vi "Parse VI XML - Splitter Style.vi"(5 "Action":T1(ring), 7 "UID":i32=83, 8 "New Style":T2 items=["Modern", "Classic", "System", "NXG"], 9 "VI XML in":string="<SL__rootObject class=\"oHExt\" uid=\"1\">\n  <root class=\"supC\" uid=\"10\">\n    <objFlags>65536</objFlags>\n    <bounds>(0, 0, 0, 0)</bounds>\n    <MouseWheelSupport>0</MouseWheelSupport>\n    <ddoList elements=\"1\">\n      <SL__arrayElement uid=\"206\"/>\n      </ddoList>\n    <paneHierarchy class=\"splitter\" uid=\"83\">\n      <objFlags>393232</objFlags>\n      <bounds>(46, 0, 434, 621)</bounds>\n      <partsList elements=\"3\">\n        <SL__arrayElement class=\"label\" uid=\"90\">\n          <objFlags>1511754</objFlags>\n          <partID>16</partID>\n          <masterPart>102</masterPart>\n          <howGrow>4108</howGrow>\n          <bounds>(133, 231, 255, 241)</bounds>\n          <image class=\"Image\">\n            <ImageResID>-9</ImageResID>\n            </image>\n          <fgColor>01000000</fgColor>\n          <bgColor>01000000</bgColor>\n          <textRec class=\"textHair\">\n            <mode>1029</mode>\n            <text>\"Splitter\"</text>\n            <bgColor>01000000</bgColor>\n            </textRec>\n          </SL__arrayElement>\n        <SL__arrayElement class=\"bigMultiCosm\" uid=\"91\">\n          <objFlags>2320</objFlags>\n          <partID>102</partID>\n          <bounds>(0, 228, 388, 234)</bounds>\n          <fgColor>00BCBCBC</fgColor>\n          <bgColor>00BCBCBC</bgColor>\n          <index>1</index>\n          <table elements=\"3\">\n            <SL__arrayElement class=\"SubCosm\">\n              <Bounds>(0, 0, 388, 6)</Bounds>\n              <FGColor>00BCBCBC</FGColor>\n              <BGColor>00BCBCBC</BGColor>\n              <Image class=\"Image\">\n                <ImageResID>-428</ImageResID>\n                </Image>\n              </SL__arrayElement>\n            <SL__arrayElement class=\"SubCosm\">\n              <Bounds>(0, 0, 388, 6)</Bounds>\n              <FGColor>00BCBCBC</FGColor>\n              <BGColor>00BCBCBC</BGColor>\n              <Image class=\"Image\">\n                <ImageResID>-11</ImageResID>\n                </Image>\n              </SL__arrayElement>\n            <SL__arrayElement class=\"SubCosm\">\n              <Bounds>(0, 0, 388, 6)</Bounds>\n              <FGColor>01000016</FGColor>\n              <BGColor>01000016</BGColor>\n              <Image class=\"Image\">\n                <ImageResID>-9</ImageResID>\n                </Image>\n              </SL__arrayElement>\n            </table>\n          </SL__arrayElement>\n        <SL__arrayElement class=\"annex\" uid=\"92\">\n          <partID>66</partID>\n          <refListLength>0</refListLength>\n          <hGrowNodeListLength>1</hGrowNodeListLength>\n          </SL__arrayElement>\n        </partsList>\n      <topOrLeft class=\"pane\" uid=\"104\">\n        <objFlags>2492464</objFlags>\n        <bounds>(0, 0, 388, 228)</bounds>\n        <partsList elements=\"6\">\n          <SL__arrayElement class=\"label\" uid=\"107\">\n            <objFlags>1511754</objFlags>\n            <partID>16</partID>\n            <masterPart>28</masterPart>\n            <howGrow>5</howGrow>\n            <bounds>(0, 0, 17, 29)</bounds>\n            <image class=\"Image\">\n              <ImageResID>-9</ImageResID>\n              </image>\n            <fgColor>01000000</fgColor>\n            <bgColor>01000000</bgColor>\n            <textRec class=\"textHair\">\n              <mode>1028</mode>\n              <text>\"Pane\"</text>\n              <bgColor>01000000</bgColor>\n              </textRec>\n            </SL__arrayElement>\n          <SL__arrayElement class=\"cosm\" uid=\"108\">\n            <objFlags>3442</objFlags>\n            <partID>39</partID>\n            <masterPart>28</masterPart>\n            <howGrow>194</howGrow>\n            <bounds>(0, 211, 371, 228)</bounds>\n            <image class=\"Image\">\n              <ImageResID>0</ImageResID>\n              </image>\n            <bgColor>00B3B3B3</bgColor>\n            </SL__arrayElement>\n          <SL__arrayElement class=\"cosm\" uid=\"109\">\n            <objFlags>3442</objFlags>\n            <partID>38</partID>\n            <masterPart>28</masterPart>\n            <howGrow>56</howGrow>\n            <bounds>(371, 0, 388, 211)</bounds>\n            <image class=\"Image\">\n              <ImageResID>0</ImageResID>\n              </image>\n            <bgColor>00B3B3B3</bgColor>\n            </SL__arrayElement>\n          <SL__arrayElement class=\"cosm\" uid=\"110\">\n            <objFlags>3443</objFlags>\n            <partID>44</partID>\n            <masterPart>28</masterPart>\n            <howGrow>10</howGrow>\n            <bounds>(371, 211, 388, 228)</bounds>\n            <image class=\"Image\">\n              <ImageResID>-365</ImageResID>\n              </image>\n            <fgColor>00B3B3B3</fgColor>\n            <bgColor>00B3B3B3</bgColor>\n            </SL__arrayElement>\n          <SL__arrayElement class=\"cosm\" uid=\"111\">\n            <objFlags>115</objFlags>\n            <partID>28</partID>\n            <howGrow>120</howGrow>\n            <bounds>(0, 0, 371, 211)</bounds>\n            <image class=\"Image\">\n              <ImageResID>-704</ImageResID>\n              </image>\n            <fgColor>00E2E2E2</fgColor>\n            <bgColor>00E2E2E2</bgColor>\n            </SL__arrayElement>\n          <SL__arrayElement class=\"annex\" uid=\"112\">\n            <partID>66</partID>\n            </SL__arrayElement>\n          </partsList>\n        <paneFlags>331089</paneFlags>\n        <minPaneSize>(1,1)</minPaneSize>\n        <docBounds>(-138, 0, 325, 232)</docBounds>\n        <zPlaneList elements=\"1\">\n          <SL__arrayElement class=\"fPDCO\" uid=\"206\">\n            <objFlags>1</objFlags>\n            <typeDesc>TypeID(1)</typeDesc>\n            <ddo class=\"stdNum\" uid=\"190\">\n              <objFlags>393217</objFlags>\n              <bounds>(0, 105, 41, 180)</bounds>\n              <partsList elements=\"8\">\n                <SL__arrayElement class=\"label\" uid=\"196\">\n                  <objFlags>1507654</objFlags>\n                  <partID>16</partID>\n                  <masterPart>9</masterPart>\n                  <howGrow>4096</howGrow>\n                  <bounds>(0, 0, 17, 22)</bounds>\n                  <image class=\"Image\">\n                    <ImageResID>-9</ImageResID>\n                    </image>\n                  <fgColor>01000000</fgColor>\n                  <bgColor>01000000</bgColor>\n                  <textRec class=\"textHair\">\n                    <flags>512</flags>\n                    <mode>17412</mode>\n                    <text>\"UID\"</text>\n                    <bgColor>01000000</bgColor>\n                    </textRec>\n                  </SL__arrayElement>\n                <SL__arrayElement class=\"numLabel\" uid=\"197\">\n                  <objFlags>264498</objFlags>\n                  <partID>10</partID>\n                  <masterPart>9</masterPart>\n                  <howGrow>240</howGrow>\n                  <bounds>(19, 2, 39, 74)</bounds>\n                  <image class=\"Image\">\n                    <ImageResID>-2002</ImageResID>\n                    </image>\n                  <fgColor>00FFFFFF</fgColor>\n                  <bgColor>00E8EBED</bgColor>\n                  <textRec class=\"textHair\">\n                    <flags>1536</flags>\n                    <mode>8389650</mode>\n                    <view>(1, 0, -2, 0)</view>\n                    <bgColor>00E8EBED</bgColor>\n                    </textRec>\n                  <format>\"%25.0f\"</format>\n                  </SL__arrayElement>\n                <SL__arrayElement class=\"bigMultiCosm\" uid=\"198\">\n                  <objFlags>6458</objFlags>\n                  <partID>2</partID>\n                  <masterPart>9</masterPart>\n                  <howGrow>2054</howGrow>\n                  <bounds>(17, 62, 28, 75)</bounds>\n                  <fgColor>002B3033</fgColor>\n                  <bgColor>00A8ABAE</bgColor>\n                  <table elements=\"2\">\n                    <SL__arrayElement class=\"SubCosm\">\n                      <Bounds>(0, 0, 11, 13)</Bounds>\n                      <FGColor>002B3033</FGColor>\n                      <BGColor>00A8ABAE</BGColor>\n                      <Image class=\"Image\">\n                        <ImageResID>-774</ImageResID>\n                        </Image>\n                      </SL__arrayElement>\n                    <SL__arrayElement class=\"SubCosm\">\n                      <Bounds>(0, 0, 11, 13)</Bounds>\n                      <FGColor>002B3033</FGColor>\n                      <BGColor>004384B7</BGColor>\n                      <Image class=\"Image\">\n                        <ImageResID>-774</ImageResID>\n                        </Image>\n                      </SL__arrayElement>\n                    </table>\n                  </SL__arrayElement>\n                <SL__arrayElement class=\"bigMultiCosm\" uid=\"199\">\n                  <objFlags>6458</objFlags>\n                  <partID>3</partID>\n                  <masterPart>9</masterPart>\n                  <howGrow>1034</howGrow>\n                  <bounds>(30, 62, 41, 75)</bounds>\n                  <fgColor>002B3033</fgColor>\n                  <bgColor>00A8ABAE</bgColor>\n                  <table elements=\"2\">\n                    <SL__arrayElement class=\"SubCosm\">\n                      <Bounds>(0, 0, 11, 13)</Bounds>\n                      <FGColor>002B3033</FGColor>\n                      <BGColor>00A8ABAE</BGColor>\n                      <Image class=\"Image\">\n                        <ImageResID>-775</ImageResID>\n                        </Image>\n                      </SL__arrayElement>\n                    <SL__arrayElement class=\"SubCosm\">\n                      <Bounds>(0, 0, 11, 13)</Bounds>\n                      <FGColor>002B3033</FGColor>\n                      <BGColor>004384B7</BGColor>\n                      <Image class=\"Image\">\n                        <ImageResID>-775</ImageResID>\n                        </Image>\n                      </SL__arrayElement>\n                    </table>\n                  </SL__arrayElement>\n                <SL__arrayElement class=\"multiCosm\" uid=\"200\">\n                  <objFlags>6458</objFlags>\n                  <partID>15</partID>\n                  <masterPart>9</masterPart>\n                  <howGrow>13</howGrow>\n                  <bounds>(22, 1, 37, 7)</bounds>\n                  <fgColor>002B3033</fgColor>\n                  <bgColor>00DBDFE2</bgColor>\n                  <table elements=\"5\">\n                    <SL__arrayElement class=\"Image\">\n                      <ImageResID>-2000</ImageResID>\n                      </SL__arrayElement>\n                    <SL__arrayElement class=\"Image\">\n                      <ImageResID>-2001</ImageResID>\n                      </SL__arrayElement>\n                    <SL__arrayElement class=\"Image\">\n                      <ImageResID>-2002</ImageResID>\n                      </SL__arrayElement>\n                    <SL__arrayElement class=\"Image\">\n                      <ImageResID>-2003</ImageResID>\n                      </SL__arrayElement>\n                    <SL__arrayElement class=\"Image\">\n                      <ImageResID>-2095</ImageResID>\n                      </SL__arrayElement>\n                    </table>\n                  </SL__arrayElement>\n                <SL__arrayElement class=\"multiCosm\" uid=\"201\">\n                  <objFlags>6462</objFlags>\n                  <partID>118</partID>\n                  <masterPart>9</masterPart>\n                  <howGrow>193</howGrow>\n                  <bounds>(18, 1, 40, 7)</bounds>\n                  <fgColor>00DBDFE2</fgColor>\n                  <bgColor>00DBDFE2</bgColor>\n                  <table elements=\"5\">\n                    <SL__arrayElement class=\"Image\">\n                      <ImageResID>-11</ImageResID>\n                      </SL__arrayElement>\n                    <SL__arrayElement class=\"Image\">\n                      <ImageResID>-11</ImageResID>\n                      </SL__arrayElement>\n                    <SL__arrayElement class=\"Image\">\n                      <ImageResID>-11</ImageResID>\n                      </SL__arrayElement>\n                    <SL__arrayElement class=\"Image\">\n                      <ImageResID>-11</ImageResID>\n                      </SL__arrayElement>\n                    <SL__arrayElement class=\"Image\">\n                      <ImageResID>-11</ImageResID>\n                      </SL__arrayElement>\n                    </table>\n                  </SL__arrayElement>\n                <SL__arrayElement class=\"cosm\" uid=\"202\">\n                  <objFlags>2327</objFlags>\n                  <partID>9</partID>\n                  <howGrow>240</howGrow>\n                  <bounds>(17, 0, 41, 75)</bounds>\n                  <image class=\"Image\">\n                    <ImageResID>-786</ImageResID>\n                    </image>\n                  <fgColor>00A8ABAE</fgColor>\n                  <bgColor>00E8EBED</bgColor>\n                  </SL__arrayElement>\n                <SL__arrayElement class=\"annex\" uid=\"203\">\n                  <partID>66</partID>\n                  <refListLength>0</refListLength>\n                  <hGrowNodeListLength>0</hGrowNodeListLength>\n                  <rsrcID>32707</rsrcID>\n                  </SL__arrayElement>\n                </partsList>\n              <typeDesc>TypeID(2)</typeDesc>\n              <MouseWheelSupport>2</MouseWheelSupport>\n              <StdNumMin>-2147483648</StdNumMin>\n              <StdNumMax>2147483647</StdNumMax>\n              <StdNumInc>0</StdNumInc>\n              </ddo>\n            <conNum>-1</conNum>\n            <termListLength>1</termListLength>\n            </SL__arrayElement>\n          </zPlaneList>\n        <image class=\"Image\">\n          <ImageResID>0</ImageResID>\n          </image>\n        </topOrLeft>\n      <botOrRight class=\"pane\" uid=\"95\">\n        <objFlags>2492464</objFlags>\n        <bounds>(0, 234, 388, 621)</bounds>\n        <partsList elements=\"6\">\n          <SL__arrayElement class=\"label\" uid=\"98\">\n            <objFlags>1511754</objFlags>\n            <partID>16</partID>\n            <masterPart>28</masterPart>\n            <howGrow>5</howGrow>\n            <bounds>(0, 0, 17, 38)</bounds>\n            <image class=\"Image\">\n              <ImageResID>-9</ImageResID>\n              </image>\n            <fgColor>01000000</fgColor>\n            <bgColor>01000000</bgColor>\n            <textRec class=\"textHair\">\n              <mode>1028</mode>\n              <text>\"Pane 2\"</text>\n              <bgColor>01000000</bgColor>\n              </textRec>\n            </SL__arrayElement>\n          <SL__arrayElement class=\"cosm\" uid=\"99\">\n            <objFlags>3442</objFlags>\n            <partID>39</partID>\n            <masterPart>28</masterPart>\n            <howGrow>194</howGrow>\n            <bounds>(0, 370, 371, 387)</bounds>\n            <image class=\"Image\">\n              <ImageResID>0</ImageResID>\n              </image>\n            <bgColor>00B3B3B3</bgColor>\n            </SL__arrayElement>\n          <SL__arrayElement class=\"cosm\" uid=\"100\">\n            <objFlags>3442</objFlags>\n            <partID>38</partID>\n            <masterPart>28</masterPart>\n            <howGrow>56</howGrow>\n            <bounds>(371, 0, 388, 370)</bounds>\n            <image class=\"Image\">\n              <ImageResID>0</ImageResID>\n              </image>\n            <bgColor>00B3B3B3</bgColor>\n            </SL__arrayElement>\n          <SL__arrayElement class=\"cosm\" uid=\"101\">\n            <objFlags>3443</objFlags>\n            <partID>44</partID>\n            <masterPart>28</masterPart>\n            <howGrow>10</howGrow>\n            <bounds>(371, 370, 388, 387)</bounds>\n            <image class=\"Image\">\n              <ImageResID>-365</ImageResID>\n              </image>\n            <fgColor>00B3B3B3</fgColor>\n            <bgColor>00B3B3B3</bgColor>\n            </SL__arrayElement>\n          <SL__arrayElement class=\"cosm\" uid=\"102\">\n            <objFlags>115</objFlags>\n            <partID>28</partID>\n            <howGrow>120</howGrow>\n            <bounds>(0, 0, 371, 370)</bounds>\n            <image class=\"Image\">\n              <ImageResID>-704</ImageResID>\n              </image>\n            <fgColor>00E2E2E2</fgColor>\n            <bgColor>00E2E2E2</bgColor>\n            </SL__arrayElement>\n          <SL__arrayElement class=\"annex\" uid=\"103\">\n            <partID>66</partID>\n            </SL__arrayElement>\n          </partsList>\n        <paneFlags>331089</paneFlags>\n        <minPaneSize>(1,1)</minPaneSize>\n        <docBounds>(-46, 0, 325, 370)</docBounds>\n        <zPlaneList elements=\"0\">\n          </zPlaneList>\n        <image class=\"Image\">\n          <ImageResID>0</ImageResID>\n          </image>\n        </botOrRight>\n      <splitterFlags>1</splitterFlags>\n      <ratio>3.671498E-1 (%x0EFBBB3E)</ratio>\n      </paneHierarchy>\n    <savedSize>(0, 0, 0, 0)</savedSize>\n    <conPane class=\"conPane\" uid=\"21\">\n      <conId>4815</conId>\n      <cons elements=\"12\">\n        </cons>\n      </conPane>\n    <keyMappingList class=\"keyMapList\" uid=\"22\">\n      </keyMappingList>\n    </root>\n  <pBounds>(46, 0, 434, 621)</pBounds>\n  <dBounds>(0, 0, 0, 0)</dBounds>\n  <origin>(435,189)</origin>\n  <instrStyle>31</instrStyle>\n  <blinkList elements=\"0\">\n    </blinkList>\n  </SL__rootObject>\n") -> (2 "Old Style":T2 items=["Modern", "Classic", "System", "NXG"], 3 "VI XML out":string="<SL__rootObject class=\"oHExt\" uid=\"1\">\n  <root class=\"supC\" uid=\"10\">\n    <objFlags>65536</objFlags>\n    <bounds>(0, 0, 0, 0)</bounds>\n    <MouseWheelSupport>0</MouseWheelSupport>\n    <ddoList elements=\"1\">\n      <SL__arrayElement uid=\"206\"/>\n      </ddoList>\n    <paneHierarchy class=\"splitter\" uid=\"83\">\n      <objFlags>393232</objFlags>\n      <bounds>(46, 0, 434, 621)</bounds>\n      <partsList elements=\"3\">\n        <SL__arrayElement class=\"label\" uid=\"90\">\n          <objFlags>1511754</objFlags>\n          <partID>16</partID>\n          <masterPart>102</masterPart>\n          <howGrow>4108</howGrow>\n          <bounds>(133, 231, 255, 241)</bounds>\n          <image class=\"Image\">\n            <ImageResID>-9</ImageResID>\n            </image>\n          <fgColor>01000000</fgColor>\n          <bgColor>01000000</bgColor>\n          <textRec class=\"textHair\">\n            <mode>1029</mode>\n            <text>\"Splitter\"</text>\n            <bgColor>01000000</bgColor>\n            </textRec>\n          </SL__arrayElement>\n        <SL__arrayElement class=\"bigMultiCosm\" uid=\"91\">\n          <objFlags>2320</objFlags>\n          <partID>102</partID>\n          <bounds>(0, 228, 388, 234)</bounds>\n          <fgColor>00BCBCBC</fgColor>\n          <bgColor>00BCBCBC</bgColor>\n          <index>1</index>\n          <table elements=\"3\">\n            <SL__arrayElement class=\"SubCosm\">\n              <Bounds>(0, 0, 388, 6)</Bounds>\n              <FGColor>00BCBCBC</FGColor>\n              <BGColor>00BCBCBC</BGColor>\n              <Image class=\"Image\">\n                <ImageResID>-428</ImageResID>\n                </Image>\n              </SL__arrayElement>\n            <SL__arrayElement class=\"SubCosm\">\n              <Bounds>(0, 0, 388, 6)</Bounds>\n              <FGColor>00BCBCBC</FGColor>\n              <BGColor>00BCBCBC</BGColor>\n              <Image class=\"Image\">\n                <ImageResID>-11</ImageResID>\n                </Image>\n              </SL__arrayElement>\n            <SL__arrayElement class=\"SubCosm\">\n              <Bounds>(0, 0, 388, 6)</Bounds>\n              <FGColor>01000016</FGColor>\n              <BGColor>01000016</BGColor>\n              <Image class=\"Image\">\n                <ImageResID>-9</ImageResID>\n                </Image>\n              </SL__arrayElement>\n            </table>\n          </SL__arrayElement>\n        <SL__arrayElement class=\"annex\" uid=\"92\">\n          <partID>66</partID>\n          <refListLength>0</refListLength>\n          <hGrowNodeListLength>1</hGrowNodeListLength>\n          </SL__arrayElement>\n        </partsList>\n      <topOrLeft class=\"pane\" uid=\"104\">\n        <objFlags>2492464</objFlags>\n        <bounds>(0, 0, 388, 228)</bounds>\n        <partsList elements=\"6\">\n          <SL__arrayElement class=\"label\" uid=\"107\">\n            <objFlags>1511754</objFlags>\n            <partID>16</partID>\n            <masterPart>28</masterPart>\n            <howGrow>5</howGrow>\n            <bounds>(0, 0, 17, 29)</bounds>\n            <image class=\"Image\">\n              <ImageResID>-9</ImageResID>\n              </image>\n            <fgColor>01000000</fgColor>\n            <bgColor>01000000</bgColor>\n            <textRec class=\"textHair\">\n              <mode>1028</mode>\n              <text>\"Pane\"</text>\n              <bgColor>01000000</bgColor>\n              </textRec>\n            </SL__arrayElement>\n          <SL__arrayElement class=\"cosm\" uid=\"108\">\n            <objFlags>3442</objFlags>\n            <partID>39</partID>\n            <masterPart>28</masterPart>\n            <howGrow>194</howGrow>\n            <bounds>(0, 211, 371, 228)</bounds>\n            <image class=\"Image\">\n              <ImageResID>0</ImageResID>\n              </image>\n            <bgColor>00B3B3B3</bgColor>\n            </SL__arrayElement>\n          <SL__arrayElement class=\"cosm\" uid=\"109\">\n            <objFlags>3442</objFlags>\n            <partID>38</partID>\n            <masterPart>28</masterPart>\n            <howGrow>56</howGrow>\n            <bounds>(371, 0, 388, 211)</bounds>\n            <image class=\"Image\">\n              <ImageResID>0</ImageResID>\n              </image>\n            <bgColor>00B3B3B3</bgColor>\n            </SL__arrayElement>\n          <SL__arrayElement class=\"cosm\" uid=\"110\">\n            <objFlags>3443</objFlags>\n            <partID>44</partID>\n            <masterPart>28</masterPart>\n            <howGrow>10</howGrow>\n            <bounds>(371, 211, 388, 228)</bounds>\n            <image class=\"Image\">\n              <ImageResID>-365</ImageResID>\n              </image>\n            <fgColor>00B3B3B3</fgColor>\n            <bgColor>00B3B3B3</bgColor>\n            </SL__arrayElement>\n          <SL__arrayElement class=\"cosm\" uid=\"111\">\n            <objFlags>115</objFlags>\n            <partID>28</partID>\n            <howGrow>120</howGrow>\n            <bounds>(0, 0, 371, 211)</bounds>\n            <image class=\"Image\">\n              <ImageResID>-704</ImageResID>\n              </image>\n            <fgColor>00E2E2E2</fgColor>\n            <bgColor>00E2E2E2</bgColor>\n            </SL__arrayElement>\n          <SL__arrayElement class=\"annex\" uid=\"112\">\n            <partID>66</partID>\n            </SL__arrayElement>\n          </partsList>\n        <paneFlags>331089</paneFlags>\n        <minPaneSize>(1,1)</minPaneSize>\n        <docBounds>(-138, 0, 325, 232)</docBounds>\n        <zPlaneList elements=\"1\">\n          <SL__arrayElement class=\"fPDCO\" uid=\"206\">\n            <objFlags>1</objFlags>\n            <typeDesc>TypeID(1)</typeDesc>\n            <ddo class=\"stdNum\" uid=\"190\">\n              <objFlags>393217</objFlags>\n              <bounds>(0, 105, 41, 180)</bounds>\n              <partsList elements=\"8\">\n                <SL__arrayElement class=\"label\" uid=\"196\">\n                  <objFlags>1507654</objFlags>\n                  <partID>16</partID>\n                  <masterPart>9</masterPart>\n                  <howGrow>4096</howGrow>\n                  <bounds>(0, 0, 17, 22)</bounds>\n                  <image class=\"Image\">\n                    <ImageResID>-9</ImageResID>\n                    </image>\n                  <fgColor>01000000</fgColor>\n                  <bgColor>01000000</bgColor>\n                  <textRec class=\"textHair\">\n                    <flags>512</flags>\n                    <mode>17412</mode>\n                    <text>\"UID\"</text>\n                    <bgColor>01000000</bgColor>\n                    </textRec>\n                  </SL__arrayElement>\n                <SL__arrayElement class=\"numLabel\" uid=\"197\">\n                  <objFlags>264498</objFlags>\n                  <partID>10</partID>\n                  <masterPart>9</masterPart>\n                  <howGrow>240</howGrow>\n                  <bounds>(19, 2, 39, 74)</bounds>\n                  <image class=\"Image\">\n                    <ImageResID>-2002</ImageResID>\n                    </image>\n                  <fgColor>00FFFFFF</fgColor>\n                  <bgColor>00E8EBED</bgColor>\n                  <textRec class=\"textHair\">\n                    <flags>1536</flags>\n                    <mode>8389650</mode>\n                    <view>(1, 0, -2, 0)</view>\n                    <bgColor>00E8EBED</bgColor>\n                    </textRec>\n                  <format>\"%25.0f\"</format>\n                  </SL__arrayElement>\n                <SL__arrayElement class=\"bigMultiCosm\" uid=\"198\">\n                  <objFlags>6458</objFlags>\n                  <partID>2</partID>\n                  <masterPart>9</masterPart>\n                  <howGrow>2054</howGrow>\n                  <bounds>(17, 62, 28, 75)</bounds>\n                  <fgColor>002B3033</fgColor>\n                  <bgColor>00A8ABAE</bgColor>\n                  <table elements=\"2\">\n                    <SL__arrayElement class=\"SubCosm\">\n                      <Bounds>(0, 0, 11, 13)</Bounds>\n                      <FGColor>002B3033</FGColor>\n                      <BGColor>00A8ABAE</BGColor>\n                      <Image class=\"Image\">\n                        <ImageResID>-774</ImageResID>\n                        </Image>\n                      </SL__arrayElement>\n                    <SL__arrayElement class=\"SubCosm\">\n                      <Bounds>(0, 0, 11, 13)</Bounds>\n                      <FGColor>002B3033</FGColor>\n                      <BGColor>004384B7</BGColor>\n                      <Image class=\"Image\">\n                        <ImageResID>-774</ImageResID>\n                        </Image>\n                      </SL__arrayElement>\n                    </table>\n                  </SL__arrayElement>\n                <SL__arrayElement class=\"bigMultiCosm\" uid=\"199\">\n                  <objFlags>6458</objFlags>\n                  <partID>3</partID>\n                  <masterPart>9</masterPart>\n                  <howGrow>1034</howGrow>\n                  <bounds>(30, 62, 41, 75)</bounds>\n                  <fgColor>002B3033</fgColor>\n                  <bgColor>00A8ABAE</bgColor>\n                  <table elements=\"2\">\n                    <SL__arrayElement class=\"SubCosm\">\n                      <Bounds>(0, 0, 11, 13)</Bounds>\n                      <FGColor>002B3033</FGColor>\n                      <BGColor>00A8ABAE</BGColor>\n                      <Image class=\"Image\">\n                        <ImageResID>-775</ImageResID>\n                        </Image>\n                      </SL__arrayElement>\n                    <SL__arrayElement class=\"SubCosm\">\n                      <Bounds>(0, 0, 11, 13)</Bounds>\n                      <FGColor>002B3033</FGColor>\n                      <BGColor>004384B7</BGColor>\n                      <Image class=\"Image\">\n                        <ImageResID>-775</ImageResID>\n                        </Image>\n                      </SL__arrayElement>\n                    </table>\n                  </SL__arrayElement>\n                <SL__arrayElement class=\"multiCosm\" uid=\"200\">\n                  <objFlags>6458</objFlags>\n                  <partID>15</partID>\n                  <masterPart>9</masterPart>\n                  <howGrow>13</howGrow>\n                  <bounds>(22, 1, 37, 7)</bounds>\n                  <fgColor>002B3033</fgColor>\n                  <bgColor>00DBDFE2</bgColor>\n                  <table elements=\"5\">\n                    <SL__arrayElement class=\"Image\">\n                      <ImageResID>-2000</ImageResID>\n                      </SL__arrayElement>\n                    <SL__arrayElement class=\"Image\">\n                      <ImageResID>-2001</ImageResID>\n                      </SL__arrayElement>\n                    <SL__arrayElement class=\"Image\">\n                      <ImageResID>-2002</ImageResID>\n                      </SL__arrayElement>\n                    <SL__arrayElement class=\"Image\">\n                      <ImageResID>-2003</ImageResID>\n                      </SL__arrayElement>\n                    <SL__arrayElement class=\"Image\">\n                      <ImageResID>-2095</ImageResID>\n                      </SL__arrayElement>\n                    </table>\n                  </SL__arrayElement>\n                <SL__arrayElement class=\"multiCosm\" uid=\"201\">\n                  <objFlags>6462</objFlags>\n                  <partID>118</partID>\n                  <masterPart>9</masterPart>\n                  <howGrow>193</howGrow>\n                  <bounds>(18, 1, 40, 7)</bounds>\n                  <fgColor>00DBDFE2</fgColor>\n                  <bgColor>00DBDFE2</bgColor>\n                  <table elements=\"5\">\n                    <SL__arrayElement class=\"Image\">\n                      <ImageResID>-11</ImageResID>\n                      </SL__arrayElement>\n                    <SL__arrayElement class=\"Image\">\n                      <ImageResID>-11</ImageResID>\n                      </SL__arrayElement>\n                    <SL__arrayElement class=\"Image\">\n                      <ImageResID>-11</ImageResID>\n                      </SL__arrayElement>\n                    <SL__arrayElement class=\"Image\">\n                      <ImageResID>-11</ImageResID>\n                      </SL__arrayElement>\n                    <SL__arrayElement class=\"Image\">\n                      <ImageResID>-11</ImageResID>\n                      </SL__arrayElement>\n                    </table>\n                  </SL__arrayElement>\n                <SL__arrayElement class=\"cosm\" uid=\"202\">\n                  <objFlags>2327</objFlags>\n                  <partID>9</partID>\n                  <howGrow>240</howGrow>\n                  <bounds>(17, 0, 41, 75)</bounds>\n                  <image class=\"Image\">\n                    <ImageResID>-786</ImageResID>\n                    </image>\n                  <fgColor>00A8ABAE</fgColor>\n                  <bgColor>00E8EBED</bgColor>\n                  </SL__arrayElement>\n                <SL__arrayElement class=\"annex\" uid=\"203\">\n                  <partID>66</partID>\n                  <refListLength>0</refListLength>\n                  <hGrowNodeListLength>0</hGrowNodeListLength>\n                  <rsrcID>32707</rsrcID>\n                  </SL__arrayElement>\n                </partsList>\n              <typeDesc>TypeID(2)</typeDesc>\n              <MouseWheelSupport>2</MouseWheelSupport>\n              <StdNumMin>-2147483648</StdNumMin>\n              <StdNumMax>2147483647</StdNumMax>\n              <StdNumInc>0</StdNumInc>\n              </ddo>\n            <conNum>-1</conNum>\n            <termListLength>1</termListLength>\n            </SL__arrayElement>\n          </zPlaneList>\n        <image class=\"Image\">\n          <ImageResID>0</ImageResID>\n          </image>\n        </topOrLeft>\n      <botOrRight class=\"pane\" uid=\"95\">\n        <objFlags>2492464</objFlags>\n        <bounds>(0, 234, 388, 621)</bounds>\n        <partsList elements=\"6\">\n          <SL__arrayElement class=\"label\" uid=\"98\">\n            <objFlags>1511754</objFlags>\n            <partID>16</partID>\n            <masterPart>28</masterPart>\n            <howGrow>5</howGrow>\n            <bounds>(0, 0, 17, 38)</bounds>\n            <image class=\"Image\">\n              <ImageResID>-9</ImageResID>\n              </image>\n            <fgColor>01000000</fgColor>\n            <bgColor>01000000</bgColor>\n            <textRec class=\"textHair\">\n              <mode>1028</mode>\n              <text>\"Pane 2\"</text>\n              <bgColor>01000000</bgColor>\n              </textRec>\n            </SL__arrayElement>\n          <SL__arrayElement class=\"cosm\" uid=\"99\">\n            <objFlags>3442</objFlags>\n            <partID>39</partID>\n            <masterPart>28</masterPart>\n            <howGrow>194</howGrow>\n            <bounds>(0, 370, 371, 387)</bounds>\n            <image class=\"Image\">\n              <ImageResID>0</ImageResID>\n              </image>\n            <bgColor>00B3B3B3</bgColor>\n            </SL__arrayElement>\n          <SL__arrayElement class=\"cosm\" uid=\"100\">\n            <objFlags>3442</objFlags>\n            <partID>38</partID>\n            <masterPart>28</masterPart>\n            <howGrow>56</howGrow>\n            <bounds>(371, 0, 388, 370)</bounds>\n            <image class=\"Image\">\n              <ImageResID>0</ImageResID>\n              </image>\n            <bgColor>00B3B3B3</bgColor>\n            </SL__arrayElement>\n          <SL__arrayElement class=\"cosm\" uid=\"101\">\n            <objFlags>3443</objFlags>\n            <partID>44</partID>\n            <masterPart>28</masterPart>\n            <howGrow>10</howGrow>\n            <bounds>(371, 370, 388, 387)</bounds>\n            <image class=\"Image\">\n              <ImageResID>-365</ImageResID>\n              </image>\n            <fgColor>00B3B3B3</fgColor>\n            <bgColor>00B3B3B3</bgColor>\n            </SL__arrayElement>\n          <SL__arrayElement class=\"cosm\" uid=\"102\">\n            <objFlags>115</objFlags>\n            <partID>28</partID>\n            <howGrow>120</howGrow>\n            <bounds>(0, 0, 371, 370)</bounds>\n            <image class=\"Image\">\n              <ImageResID>-704</ImageResID>\n              </image>\n            <fgColor>00E2E2E2</fgColor>\n            <bgColor>00E2E2E2</bgColor>\n            </SL__arrayElement>\n          <SL__arrayElement class=\"annex\" uid=\"103\">\n            <partID>66</partID>\n            </SL__arrayElement>\n          </partsList>\n        <paneFlags>331089</paneFlags>\n        <minPaneSize>(1,1)</minPaneSize>\n        <docBounds>(-46, 0, 325, 370)</docBounds>\n        <zPlaneList elements=\"0\">\n          </zPlaneList>\n        <image class=\"Image\">\n          <ImageResID>0</ImageResID>\n          </image>\n        </botOrRight>\n      <splitterFlags>1</splitterFlags>\n      <ratio>3.671498E-1 (%x0EFBBB3E)</ratio>\n      </paneHierarchy>\n    <savedSize>(0, 0, 0, 0)</savedSize>\n    <conPane class=\"conPane\" uid=\"21\">\n      <conId>4815</conId>\n      <cons elements=\"12\">\n        </cons>\n      </conPane>\n    <keyMappingList class=\"keyMapList\" uid=\"22\">\n      </keyMappingList>\n    </root>\n  <pBounds>(46, 0, 434, 621)</pBounds>\n  <dBounds>(0, 0, 0, 0)</dBounds>\n  <origin>(435,189)</origin>\n  <instrStyle>31</instrStyle>\n  <blinkList elements=\"0\">\n    </blinkList>\n  </SL__rootObject>\n")   [LabVIEW 2020, in "Splitter.lvclass"]
uses:
  Splitter.lvclass
  Typedefs/Splitter Style--Enum.ctl
  Splitter.lvclass/Splitter.ctl
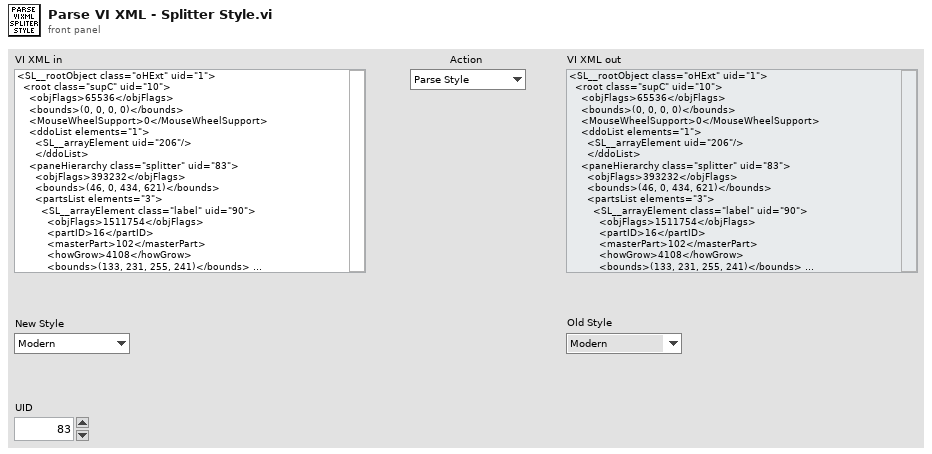
[diagram p1: front panel]
types:
  T1 = enum16{"Parse Style", "Update Style", "Store XML"}
  T2 = typedef "Splitter Style--Enum.ctl" = u16
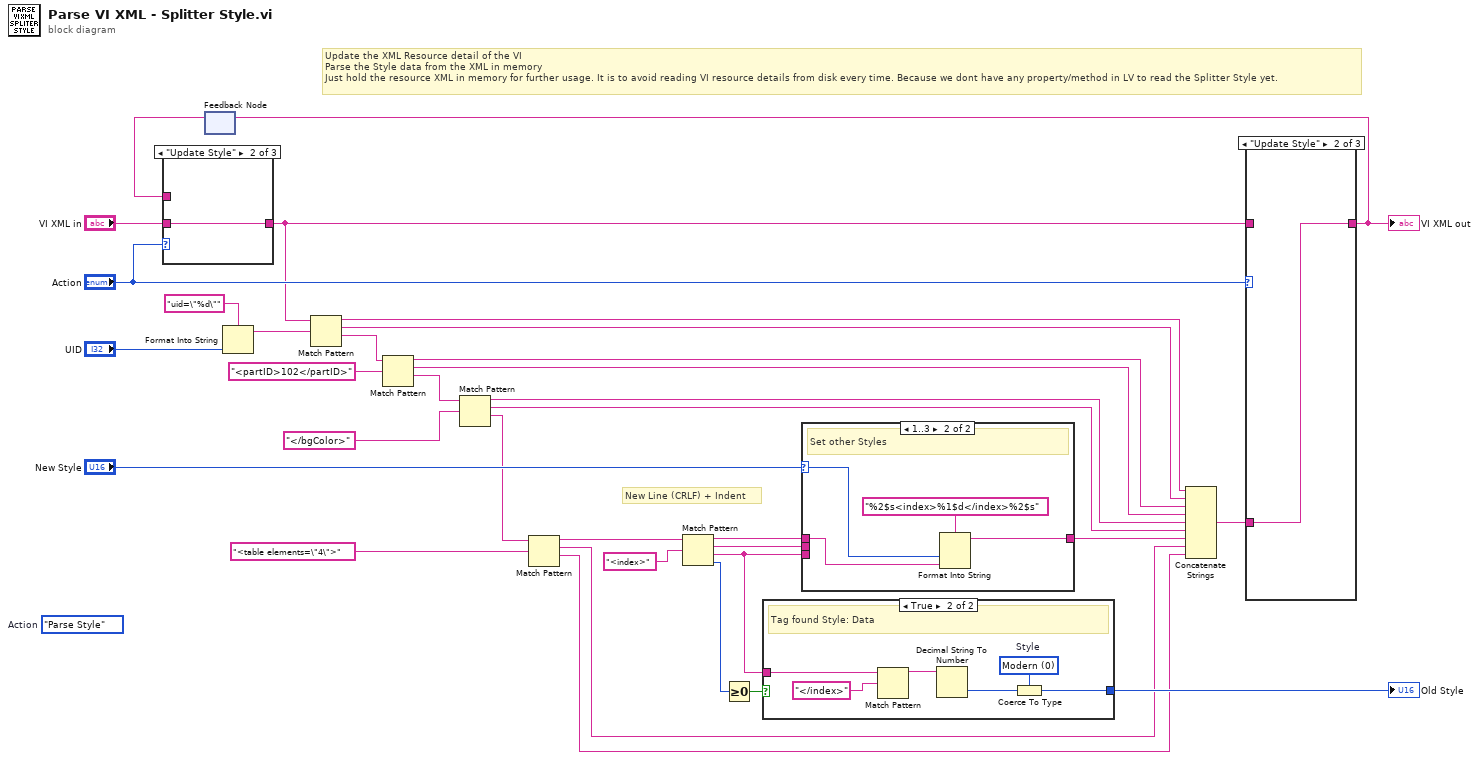
[diagram p0: block diagram]
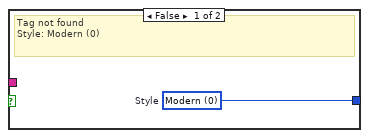
[diagram p7: hidden frame]
diagram:
  (unwired) T1."Parse Style"  # Action
  # "New Line (CRLF) + Indent"
  # "Update the XML Resource detail of the VI\nParse the Style data from the XML in memory\nJust hold the resource XML in memory for further usage. It is to avoid reading VI resource details from disk every time. Because we dont have any property/method in LV to read the Splitter Style yet."
  n1 = feedback #1() -> (w5:string)  [unwired: 1 in]
  n2 = case shown="\"Update Style\"" "Action" {
    tunnel: "VI XML in" -> [_ w35 w36]
    tunnel: w5 -> [w34 _ _]
    tunnel: [w34 w35 w36] -> w1
    frame "Parse Style" {
    }
    frame "Update Style" {
    }
    frame "Store XML" {
    }
  }
  n3 = Format Into String(format string="uid=\"%d\"", "UID") -> (resulting string=w29:string)  [unwired: 2 in, 1 out]
  n4 = Match Pattern(string=w1, regular expression=w29) -> (before substring=w21:string, match substring=w22:string, after substring=w10:string)  [unwired: 1 in, 1 out]
  n5 = Match Pattern(string=w10, regular expression="<partID>102</partID>" ("format string")) -> (before substring=w8:string, match substring=w7:string, after substring=w9:string)  [unwired: 1 in, 1 out]
  n6 = Match Pattern(string=w9, regular expression="</bgColor>" ("format string")) -> (before substring=w23:string, match substring=w24:string, after substring=w27:string)  [unwired: 1 in, 1 out]
  n7 = Match Pattern(string=w27, regular expression="<table elements=\"4\">" ("format string")) -> (before substring=w19:string, match substring=w25:string, after substring=w20:string)  [unwired: 1 in, 1 out]
  n8 = Match Pattern(string=w19, regular expression="<index>" ("format string")) -> (before substring=w15:string, match substring=w13:string, after substring=w12:string, offset past match=w17:i32)  [unwired: 1 in]
  n9 = Greater Or Equal To 0?(x=w17) -> (x >= 0?=w16:bool)
  n10 = case shown="True" w16 {
    tunnel: w12 -> [_ w42]
    tunnel: [w37 w39] -> w32
    frame False {
      w37 = T2 0 items=["Modern", "Classic", "System", "NXG"]  # Style
      # "Tag not found\nStyle: Modern (0)"
    }
    frame True {
      w38 = T2 0 items=["Modern", "Classic", "System", "NXG"]  # Style
      # "Tag found Style: Data"
      n11 = Match Pattern(string=w42, regular expression="</index>" ("format string")) -> (before substring=w41:string)  [unwired: 1 in, 3 out]
      n12 = Decimal String To Number(string=w41) -> (number=w40:i32)  [unwired: 2 in, 1 out]
      n13 = Coerce To Type(0:w40, 1:w38) -> (2:w39:T2)
    }
  }
  "Old Style" <- w32
  n14 = case shown="1..3" "New Style" {
    selector: "New Style" -> [_ w45]
    tunnel: [w44 w47] -> w14
    tunnel: w15 -> [w44 w46]
    tunnel: w13 -> [_ _]
    tunnel: w12 -> [_ _]
    frame 0, Default {
      # "Set Style: Modern"
    }
    frame 1..3 {
      # "Set other Styles"
      n15 = Format Into String(format string="%2$s<index>%1$d</index>%2$s", w45, w46) -> (resulting string=w47:string)  [unwired: 2 in, 1 out]
    }
  }
  n16 = Concatenate Strings(w21, w22, w8, w7, w23, w24, w14, w25, w20) -> (w3:string)
  n17 = case shown="\"Update Style\"" "Action" {
    tunnel: w3 -> [_ w50 _]
    tunnel: [w49 w50 w51] -> w2
    tunnel: w1 -> [w49 _ w51]
    frame "Parse Style" {
    }
    frame "Update Style" {
    }
    frame "Store XML" {
    }
  }
  "VI XML out" <- w2
  n18 = feedback-in #1(w2) -> ()
